vi "Read statvfs.vi"(8 "error in (no error)":errorcluster, 11 "Filesystem Statistics in":refnum<class "Filesystem Statistics.lvclass">) -> (0 "error out":errorcluster, 2 "statvfs@openssh.com reply":T1 {"f_flag" format="%x"; "f_fsid" format="%x"}, 3 "Filesystem Statistics out":refnum<class "Filesystem Statistics.lvclass">)   [LabVIEW 2020, in "NI_SFTP.lvlib" / "Filesystem Statistics.lvclass"]
doc: "Reads the statvfs object contained in this Filesystem Statistics object. This is the low-level information used to calculate all other properties."
uses:
  <vilib>/net/SFTP/Filesystem Statistics/Filesystem Statistics.lvclass
  <vilib>/net/SFTP/API/Support/statvfs info.ctl
  <vilib>/net/SFTP/Filesystem Statistics/Filesystem Statistics.lvclass/Filesystem Statistics.ctl
  <vilib>/net/SFTP/NI_SFTP.lvlib
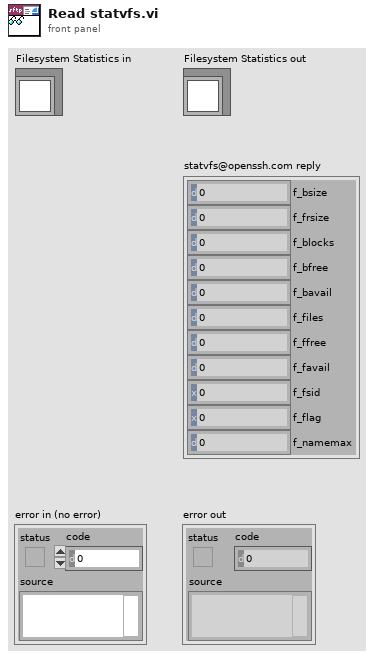
[diagram p1: front panel]
types:
  T1 = typedef "NI_SFTP.lvlib/statvfs info.ctl" = cluster{"f_bsize":u64, "f_frsize":u64, "f_blocks":u64, "f_bfree":u64, "f_bavail":u64, "f_files":u64, "f_ffree":u64, "f_favail":u64, "f_fsid":u64, "f_flag":u64, "f_namemax":u64}
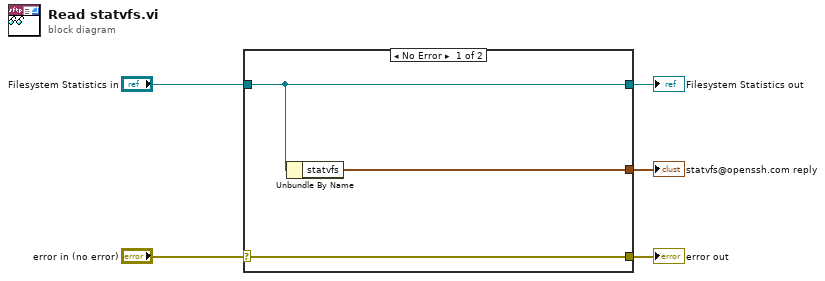
[diagram p0: block diagram]
diagram:
  n1 = case shown="No Error" "error in (no error)" {
    selector: "error in (no error)" -> [w8 w9]
    tunnel: [w8 w9] -> w4
    tunnel: [w7 w10] -> w2
    tunnel: "Filesystem Statistics in" -> [w7 w10]
    tunnel: [w6 _] -> w1
    frame No Error {
      n2 = Unbundle By Name(w7) -> ("statvfs"=w6:T1)
    }
    frame Error {
    }
  }
  "error out" <- w4
  "Filesystem Statistics out" <- w2
  "statvfs@openssh.com reply" <- w1
